vi "Gaussian surface with offset fit For g.vi"() -> ()   [LabVIEW 2013]
doc: "Demonstrates fitting a 2D surface using the Nonlinear Curve Fit VI. Shows use of the curve fitting interface to implement a live update of a graph during the fitting process. Also demonstrates the use of analytic derivatives in the model function."
uses:
  <vilib>/Native 3D Graph/xcontrol/3DPC_SurfacePlot.xctl
  <vilib>/gmath/NumericalOptimization/Nonlinear Curve Fit LM.vi
  <vilib>/gmath/NI_Gmath.lvlib
panel:
  out "Best Fits":dbl[](array[numeric])
  in  "Parameters":dbl[](array[numeric])=[2.0, 0.3, 0.06, 0.7, 0.14, 1.0]
  in  "Tab Control":enum32{"Graph", "Equation"}(tab)
  out "3D Surface Graph":refnum<class "Base Datatype.lvclass">[](xcontrol)
  in  "Fit data?":bool
  in  "Stop":bool
  in  "num Y samples":i32=50
  in  "num X samples":i32=100
  out "#function calls":i32
  out "residue":dbl
  in  "noise sigma":dbl=0.05
  # "Overview: Demonstrates fitting a 2D surface using the Nonlinear Curve Fit VI.  \nRequirements: LabVIEW Full Development System\nInstructions:\n1. Run the VI.\n2. Click the Fit Data button to perform a fit on the 2D surface. Observe the intermediate steps as the fit is calculated.\n3. Click Stop to stop the VI."
  # "Amplitude"
  # "m1 (Mean 1)"
  # "Sigma 1"
  # "m2 (Mean 2)"
  # "Sigma 2"
  # "Offset"
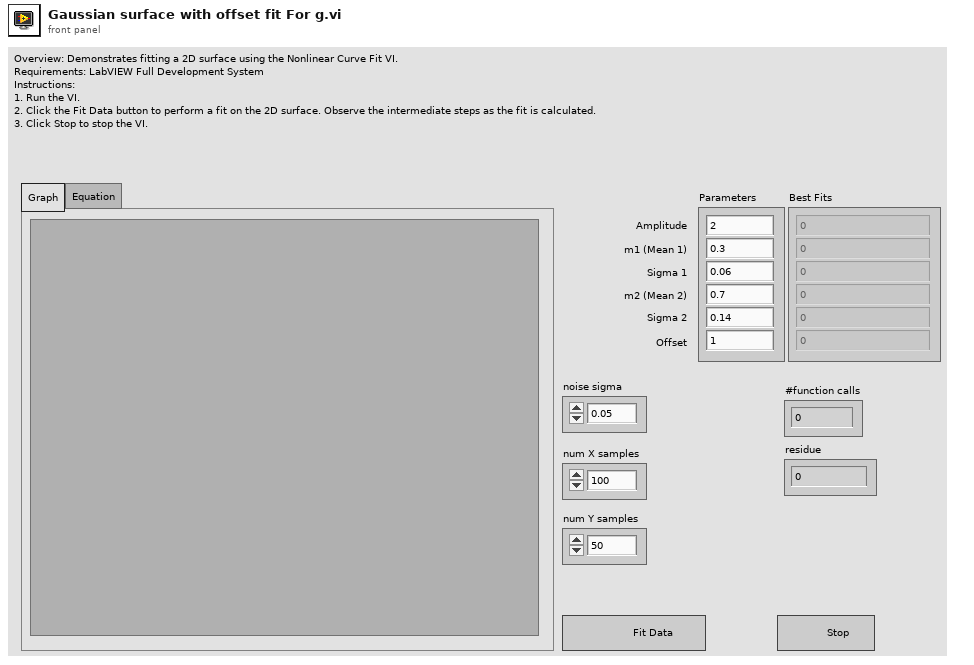
[diagram p1: front panel]
types:
  T1 = cluster{"3D Surface Graph":refnum<vi>, "num X samples":i32, "num Y samples":i32}
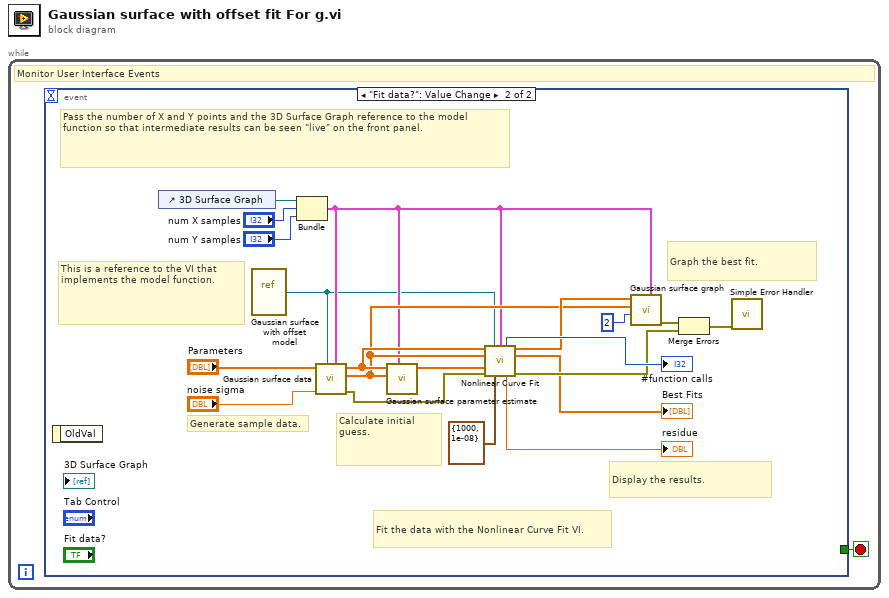
[diagram p0: block diagram]
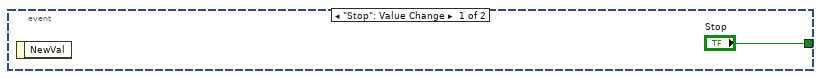
[diagram p2: hidden frame]
diagram:
  n1 = while {
    stop <- w1 stop-if-true
    # "Monitor User Interface Events"
    n2 = event shown="[1] \"Fit data?\": Value Change" {
      selector: _ -> [_ _]
      dyn-events: _ -> [_ _]
      timeout: _ -> [_ _]
      tunnel: ["Stop" _] -> w1
      event "Stop": Value Change {
        n3 = event-data() -> ()  [unwired: 2 out]
      }
      event "Fit data?": Value Change {
        # "Graph the best fit."
        # "Pass the number of X and Y points and the 3D Surface Graph reference to the model function so that intermediate results can be seen \"live\" on the front panel."
        # "Fit the data with the Nonlinear Curve Fit VI."
        # "Display the results."
        # "Calculate initial guess."
        # "This is a reference to the VI that implements the model function."
        # "Generate sample data."
        n4 = event-data() -> ()  [unwired: 2 out]
        n5 = control-ref of="3D Surface Graph"() -> (w13:refnum<vi>)
        n6 = vi-ref "Gaussian surface with offset model.vi"() -> (w5:refnum<vi>)
        n7 = Bundle("3D Surface Graph"=w13, "num X samples"="num X samples", "num Y samples"="num Y samples") -> (w10:T1)  [unwired: 1 out]
        n8 = call "Gaussian surface data.vi"("output cluster"=w10, "VI Refnum"=w5, "noise sigma"="noise sigma", "a"="Parameters") -> ("error out"=w9:errorcluster, "X"=w11:dbl[], "Noisy 2D Gaussian surface data"=w12:dbl[])  [unwired: 4 in, 1 out]
        n9 = call "Gaussian surface parameter estimate.vi"("output cluster"=w10, "X"=w11, "Y"=w12) -> ("estimated parameters"=w19:dbl[])  [unwired: 8 out]
        n10 = call-poly <vilib>:"Nonlinear Curve Fit.vi"("Y"=w12, "f(x,a)"=w5, "data"=w10, "X"=w11, "initial parameters"=w19, "error in (no error)"=w9, "termination"=cluster{"max iteration":i32, "tolerance":dbl} {"max iteration"=1000, "tolerance"=1e-08}) -> ("number of function calls"=→"#function calls":i32, "best nonlinear fit"=w14:dbl[], "best fit parameters"=→"Best Fits":dbl[], "residue"=→"residue":dbl, "error out"=w8:errorcluster)  [unwired: 1 in, 3 out]
        n11 = call "Gaussian surface graph.vi"("output cluster"=w10, "plot number (1)"=2, "X"=w11, "Y"=w14) -> ("error out"=w7:errorcluster)  [unwired: 1 in, 6 out]
        n12 = Merge Errors(w7, w8) -> (w6:errorcluster)
        n13 = call <vilib>:"Simple Error Handler.vi"("error in (no error)"=w6) -> ()  [unwired: 4 in, 5 out]
      }
    }
  }
